vi "plcHMI_scope.vi"() -> ()   [LabVIEW 2020]
doc: "ADS continuos synchronous write example using base blocks. \n\nThe client writes data synchronously and does wait for the respose from server."
uses:
  Agilent/AgilentTotalCluster.ctl
  Agilent/AgilentControl.ctl
  Agilent/Channel Config.ctl
  <vilib>/Platform/TimedLoop/XDataNode/timing_clust.ctl
  <vilib>/Platform/TimedLoop/XDataNode/nitl_modes.ctl
  <vilib>/Platform/TimedLoop/XDataNode/wakeup.ctl
  <vilib>/Platform/TimedLoop/XDataNode/XDataNode.xnode
  <vilib>/Platform/TimedLoop/XDataNode/XDNodeRunTimeDep.lvlib
panel:
  in  "Tab Control":T1(tab)
  in  "Symbol file path - MUST BE ENTERED\nLoad \"ADS Write AND Read Symbols REV X.X.xml\"":path
  in  "EXIT HMI":bool caption="STOP HMI\nEXIT HMI"
  in  "CH4 Vertical Units":string(combo)="V"
  in  "CH4 Vertical Units/div":dbl=2.0
  in  "Toggle Scope Scale":bool
  in  "CH1 Vertical Units/div":dbl=2.0
  in  "CH1 Vertical Units":string(combo)="V"
  in  "Horizontal Units":enum16{"us", "ms", "s"}(ring)
  in  "Horizontal Units/div":dbl=200.0
  out "Download":bool
  in  "Single":bool
  in  "Stop":bool
  in  "Agilent Array":T2[](array[typedef])
  in  "C:\\HVTest\\Local_Cap_Log_Scope (.xlsx)":path
  in  "Process Step":i32
  # "CONFIGURATION"
  # "Press STOP HMI instead of\nLabView Abort Execution"
  # "INPUT VARIABLES - For TDK Lambda 802L\nMust be written to before START"
  # "FAULT STATUSES"
  # "Set to -1 for automated\nfull charge to setpoint"
  # "MANUAL CONTROLS"
  # "Does not record during \"wait\" and appends to data file. Must be named with .xlsx"
  # "HV Switch Configuration"
  # "Records during \"Test Running.\" Must be named with .xlsx"
  # "Control Sys Faults"
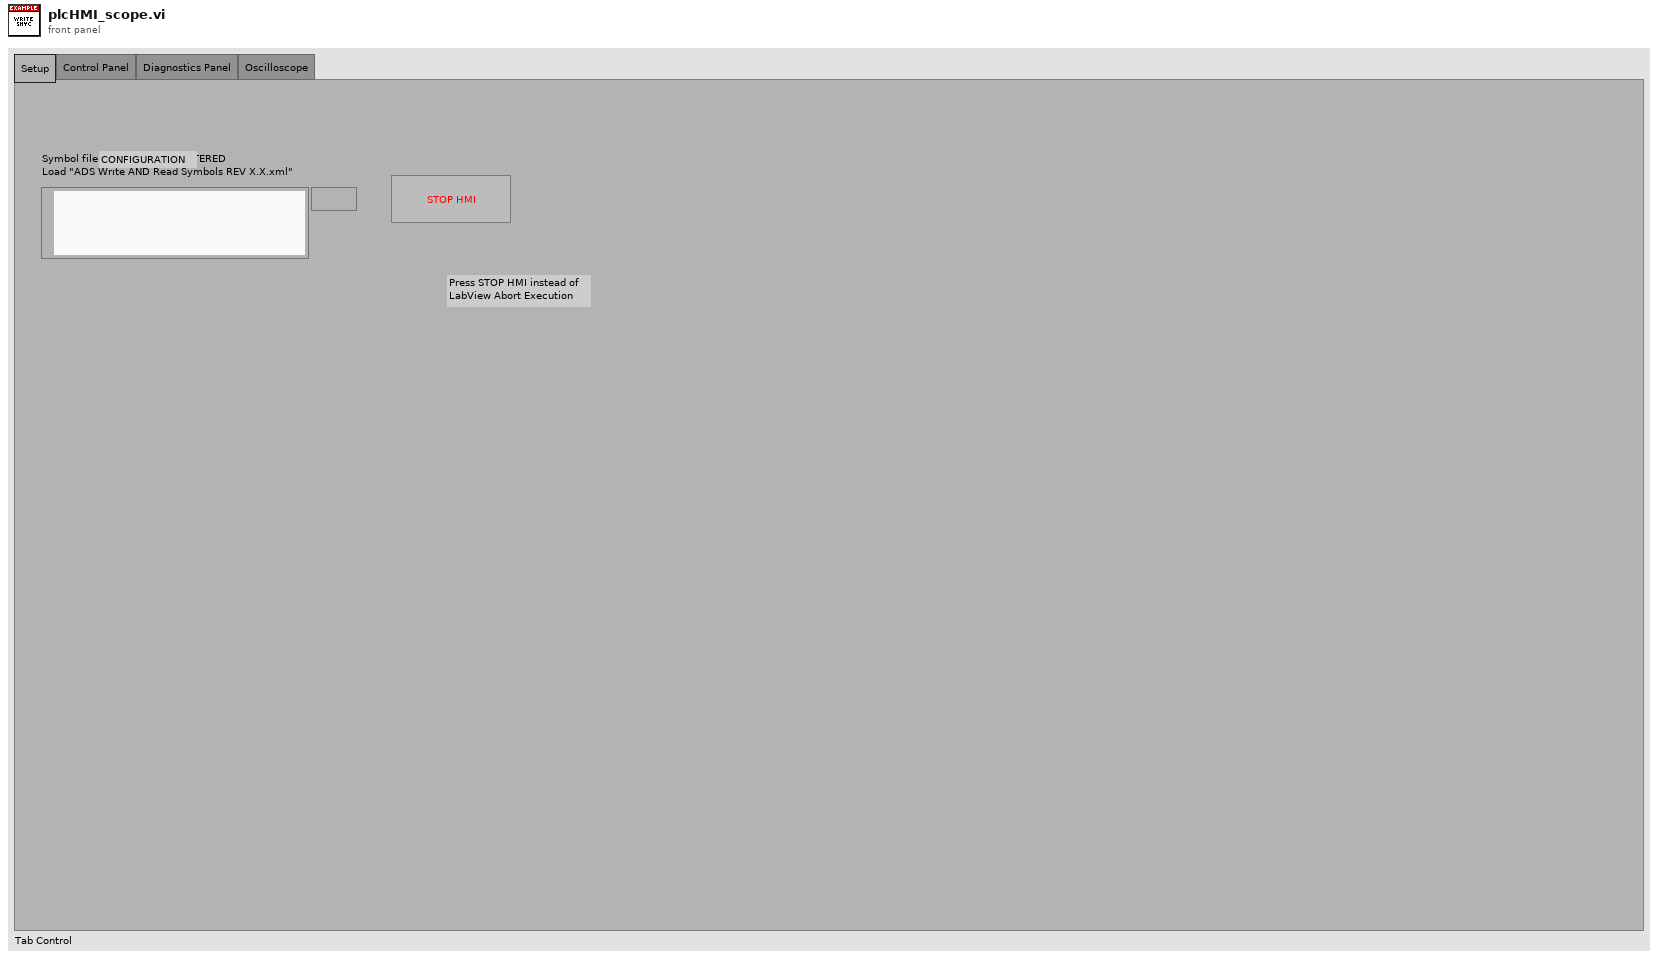
[diagram p1: front panel]
types:
  T1 = enum32{"Setup", "Control Panel", "Diagnostics Panel", "Oscilloscope"}
  T2 = typedef "AgilentTotalCluster.ctl" = cluster{"Agilent Graph":waveform(dbl)[], "Agilent Control":T3, "Agilent Setup Error":errorcluster, "Agilent Present":bool, "Enabled":bool}
  T3 = typedef "AgilentControl.ctl" = cluster{"Trig?":bool, "VISA session":refnum<visa-resource-name>, "Setup to Load":string, "Timeout (ms)":u32, "Desired Samp":enum32{"100", "250", "500", "1000", "2000", "5000", "10000", "20000", "50000", "100000", "200000", "500000", "1000000", "2000000", "4000000", "8000000"}, "Captured Samp":i32, "Desired Channels":T4[]}
  T4 = typedef "Channel Config.ctl" = cluster{"Chan Index":enum16{"Channel1", "Channel2", "Channel3", "Channel4", "MATH"}, "Name":string, "Samples":i32}
  T5 = typedef "XDNodeRunTimeDep.lvlib/timing_clust.ctl" = cluster{"Expected End [f-1]":u64, "Actual End [f-1]":u64, "Finished Late? [f-1]":bool, "Expected End [i-1]":u64, "Actual End [i-1]":u64, "Finished Late? [i-1]":bool, "Expected Start [i]":u64, "Actual Start [i]":u64, "Expected Start [f]":u64, "Actual Start [f]":u64, "Source Name":string, "Structure Name":string, "Period":i64, "Deadline":i64, "Offset":i64, "Start":i64, "Priority":i32, "Timeout":i32, "Mode":T6, "Wakeup Reason":T7, "Error":errorcluster, "Source Type":string, "Secondary Source Type":string, "Global End Time":u64, "Global Start Time":u64, "Frame Duration":u64, "Iteration Duration":u64, "Assigned CPU":i32, "I/O Scan Engine Mode":u32}
  T6 = typedef "XDNodeRunTimeDep.lvlib/nitl_modes.ctl" = enum32{"No Change", "Process missed periods, maintain original phase", "Discard missed periods, maintain original phase", "Process missed periods, ignore original phase", "Discard missed periods, ignore original phase"}
  T7 = typedef "XDNodeRunTimeDep.lvlib/wakeup.ctl" = enum32{"Normal", "Aborted", "Asynchronous wakeup", "Timing source error", "Timed loop error", "Timeout"}
  T8 = cluster{"Agilent Array[0]":T2, "Agilent Array[1]":T2, "Agilent Array[2]":T2, "Agilent Array[3]":T2, "Agilent Array[4]":T2, "Agilent Array[5]":T2, "Agilent Array[6]":T2, "Agilent Array[7]":T2, "Agilent Array[8]":T2}
  T9 = enum32{"100", "250", "500", "1000", "2000", "5000", "10000", "20000", "50000", "100000", "200000", "500000", "1000000", "2000000", "4000000", "8000000"}
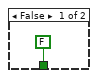
[diagram p2: hidden frame]
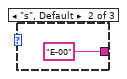
[diagram p5: hidden frame]
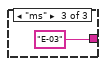
[diagram p6: hidden frame]
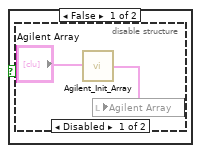
[diagram p7: hidden frame]
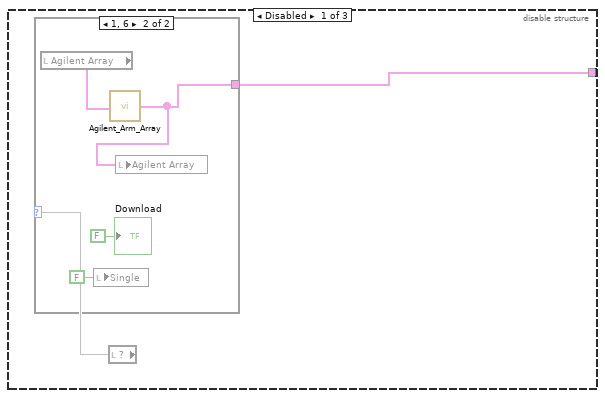
[diagram p11: hidden frame]
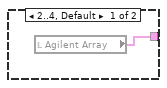
[diagram p12: hidden frame]
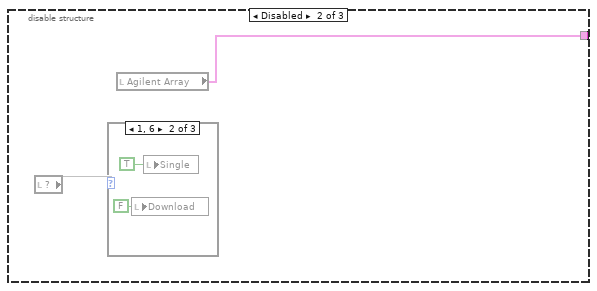
[diagram p13: hidden frame]
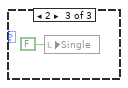
[diagram p15: hidden frame]
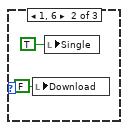
[diagram p17: hidden frame]
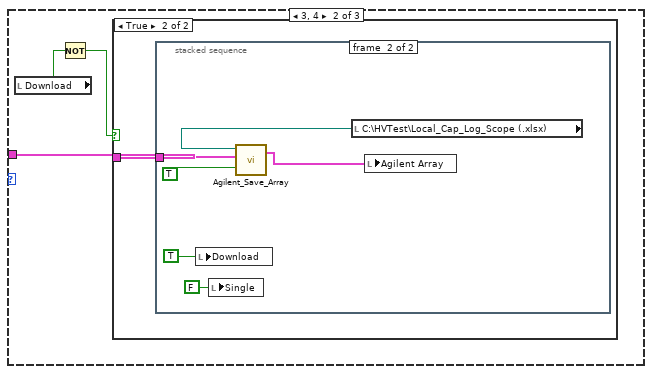
[diagram p19: hidden frame]
diagram:
  # "Symbol Interface"
  n1 = disable-structure shown="Enabled" {
    disable-tunnel: [w5 _] -> _
    disable-tunnel: [w4 w6] -> _
    frame Disabled {
      # "Using Symbol Interface"
      n2 = call <userlib>:"Symbol Interface.vi"() -> ("PortInfo"=w4:string, "error out"=w5:errorcluster)  [unwired: 14 in]
    }
    frame Enabled {
      # "Using Symbol File"
      n3 = Path To String(path="Symbol file path - MUST BE ENTERED\nLoad \"ADS Write AND Read Symbols REV X.X.xml\"") -> (string=w6:string)
    }
  }
  n4 = node-c288(10) -> (w3:T5)  [unwired: 3 in]
  n5 = timed-loop {
    timing: w3 -> [_]
    timing-out: [_] -> w2
    stop <- "EXIT HMI" stop-if-true
    n6 = node-c288() -> ()  [unwired: 1 in, 1 out]
    n7 = disable-structure shown="Enabled" {
      frame Enabled {
        n8 = flat-sequence {
          tunnel: [w65] -> w9
          tunnel: w9 -> [w84]
          frame #0 {
            n9 = disable-structure shown="Enabled" {
              frame Enabled {
                n10 = feedback #1(TRUE) -> (w11:bool)
                n11 = And(x=TRUE, y=w11) -> (x .and. y?=w14:bool)
                n12 = case shown="True" w14 {
                  tunnel: [FALSE FALSE] -> w12
                  frame False {
                  }
                  frame True {
                    n13 = local read "Agilent Array"() -> (w17:T2[])
                    n14 = call "Agilent_Init_Array.vi"("Agilent Array In"=w17) -> ("Agilent Array Out"=w18:T2[])
                    n15 = call "Agilent_Arm_Array.vi"("Agilent Array In"=w18) -> ("Agilent Array Out"=w16:T2[])
                    n16 = local write "Agilent Array"(w16) -> ()
                  }
                }
                n17 = feedback-in #1(w12) -> ()
              }
              frame Disabled {
              }
            }
          }
          frame #1 {
            n18 = case shown="True" "Toggle Scope Scale" {
              frame False {
              }
              frame True {
                n19 = Number To Decimal String(number="CH4 Vertical Units/div") -> (decimal integer string=w24:string)  [unwired: 1 in]
                n20 = Number To Decimal String(number="Horizontal Units/div") -> (decimal integer string=w32:string)  [unwired: 1 in]
                n21 = Number To Decimal String(number="CH1 Vertical Units/div") -> (decimal integer string=w30:string)  [unwired: 1 in]
                n22 = case shown="\"us\"" "Horizontal Units" {
                  tunnel: ["E-06" "E-00" "E-03"] -> w41
                  frame "us" {
                  }
                  frame "s", Default {
                  }
                  frame "ms" {
                  }
                }
                n23 = Concatenate Strings(":CHAN4:SCAL " ("write buffer"), w24, "CH4 Vertical Units") -> (w23:string)
                n24 = Concatenate Strings(":CHAN1:SCAL " ("write buffer"), w30, "CH1 Vertical Units") -> (w37:string)
                n25 = Concatenate Strings(":TIM:SCAL " ("write buffer"), w32, w41) -> (w40:string)
                n26 = VISA Open(VISA resource name=refnum<visa-resource-name> "HV_Test_Scope") -> (VISA resource name=w35:refnum<visa-resource-name>, error out=w36:errorcluster)  [unwired: 4 in]
                n27 = VISA Write(VISA resource name=w35, write buffer=w40, error in (no error)=w36) -> (VISA resource name out=w44:refnum<visa-resource-name>, error out=w43:errorcluster)  [unwired: 1 out]
                n28 = VISA Write(VISA resource name=w44, write buffer=w37, error in (no error)=w43) -> (VISA resource name out=w29:refnum<visa-resource-name>, error out=w27:errorcluster)  [unwired: 1 out]
                n29 = VISA Write(VISA resource name=w29, write buffer=w23, error in (no error)=w27) -> (VISA resource name out=w28:refnum<visa-resource-name>, error out=w26:errorcluster)  [unwired: 1 out]
                n30 = VISA Close(VISA resource name=w28, error in (no error)=w26) -> ()  [unwired: 1 out]
              }
            }
          }
          frame #2 {
            n31 = disable-structure shown="Enabled" {
              frame Enabled {
                n32 = case shown="True" "Stop" {
                  frame False {
                    n33 = disable-structure shown="Disabled" {
                      frame Disabled {
                        n34 = call "Agilent_Init_Array.vi"("Agilent Array In"="Agilent Array") -> ("Agilent Array Out"=w51:T2[])
                        n35 = local write "Agilent Array"(w51) -> ()
                      }
                      frame Enabled {
                      }
                    }
                  }
                  frame True {
                    n36 = VISA Open(VISA resource name=refnum<visa-resource-name> "HV_Test_Scope") -> (VISA resource name=w57:refnum<visa-resource-name>, error out=w58:errorcluster)  [unwired: 4 in]
                    n37 = VISA Write(VISA resource name=w57, write buffer=":STOP", error in (no error)=w58) -> (VISA resource name out=w55:refnum<visa-resource-name>, error out=w56:errorcluster)  [unwired: 1 out]
                    n38 = VISA Close(VISA resource name=w55, error in (no error)=w56) -> ()  [unwired: 1 out]
                  }
                }
              }
              frame Disabled {
              }
            }
            n39 = case shown="True" "Single" {
              frame False {
              }
              frame True {
                n40 = VISA Open(VISA resource name=refnum<visa-resource-name> "HV_Test_Scope") -> (VISA resource name=w63:refnum<visa-resource-name>, error out=w64:errorcluster)  [unwired: 4 in]
                n41 = VISA Write(VISA resource name=w63, write buffer=":SINGLE", error in (no error)=w64) -> (VISA resource name out=w61:refnum<visa-resource-name>, error out=w62:errorcluster)  [unwired: 1 out]
                n42 = VISA Close(VISA resource name=w61, error in (no error)=w62) -> ()  [unwired: 1 out]
              }
            }
          }
          frame #3 {
            n43 = disable-structure shown="Enabled" {
              disable-tunnel: [w67 w74 w79] -> w65
              frame Disabled {
                n44 = local read item#-1() -> (w66)
                n45 = case shown="1, 6" w66 {
                  tunnel: [w68 w72] -> w67
                  frame 2..4, Default {
                    n46 = local read "Agilent Array"() -> (w68:T2[])
                  }
                  frame 1, 6 {
                    n47 = local read "Agilent Array"() -> (w69:T2[])
                    n48 = local write "Single"(FALSE ("Single")) -> ()
                    n49 = call "Agilent_Arm_Array.vi"("Agilent Array In"=w69) -> ("Agilent Array Out"=w72:T2[])
                    n50 = local write "Agilent Array"(w72) -> ()
                    "Download" <- FALSE ("Downloading")
                  }
                }
              }
              frame Disabled {
                n51 = local read item#-1() -> (w73)
                n52 = case shown="1, 6" w73 {
                  frame 0, Default {
                  }
                  frame 1, 6 {
                    n53 = local write "Download"(FALSE ("Download")) -> ()
                    n54 = local write "Single"(TRUE ("Single")) -> ()
                  }
                  frame 2 {
                    n55 = local write "Single"(FALSE ("Single")) -> ()
                  }
                }
                n56 = local read "Agilent Array"() -> (w74:T2[])
              }
              frame Enabled {
                n57 = case shown="2, 7" "Process Step" {
                  frame 0, Default {
                  }
                  frame 1, 6 {
                    n58 = local write "Download"(FALSE ("Download")) -> ()
                    n59 = local write "Single"(TRUE ("Single")) -> ()
                  }
                  frame 2, 7 {
                    n60 = local write "Single"(FALSE ("Single")) -> ()
                  }
                }
                n61 = local read "Agilent Array"() -> (w79:T2[])
              }
            }
          }
          frame #4 {
            n62 = local read "Process Step"() -> (w83:i32)
            n63 = case shown="0" w83 {
              tunnel: w84 -> [_ w87 w100]
              frame Default {
              }
              frame 3, 4 {
                n64 = local read "Download"() -> (w86:bool)
                n65 = Not(x=w86) -> (.not. x?=w85:bool)
                n66 = case shown="True" w85 {
                  tunnel: w87 -> [_ w88]
                  frame False {
                  }
                  frame True {
                    n67 = stacked-sequence {
                      tunnel: w88 -> [_ w98]
                      frame #0 {
                        n68 = local read "Agilent Array"() -> (w92:T2[])
                        n69 = Array To Cluster(array=w92) -> (cluster=w91:T8)
                        n70 = Unbundle By Name(w91) -> ("Agilent Array[0].Agilent Control.Desired Samp"=w89:T9)
                        n71 = call "GF_SetRecordLengthProperly.vi"("Num Samples"=w89, "VISA resource name"=refnum<visa-resource-name> "HV_Test_Scope") -> ()  [unwired: 1 in, 2 out]
                      }
                      frame #1 {
                        n72 = local write "Download"(TRUE ("Downloading")) -> ()
                        n73 = local write "Single"(FALSE ("Single")) -> ()
                        n74 = local read "C:\\HVTest\\Local_Cap_Log_Scope (.xlsx)"() -> (w93:path)
                        n75 = call "Agilent_Save_Array.vi"("Agilent Download"=TRUE, "Agilent Array In"=w98, "File Path"=w93) -> ("Agilent Array Out"=w96:T2[])  [unwired: 1 in, 1 out]
                        n76 = local write "Agilent Array"(w96) -> ()
                      }
                    }
                  }
                }
              }
              frame 0 {
                n77 = local read "Process Step"() -> (w99:i32)
                n78 = case shown="1" w99 {
                  tunnel: w100 -> [_ w103]
                  frame 0, Default {
                  }
                  frame 1 {
                    n79 = local read "Download"() -> (w102:bool)
                    n80 = Not(x=w102) -> (.not. x?=w101:bool)
                    n81 = case shown="True" w101 {
                      tunnel: w103 -> [_ w104]
                      frame False {
                      }
                      frame True {
                        n82 = stacked-sequence {
                          tunnel: w104 -> [_ w114]
                          frame #0 {
                            n83 = local read "Agilent Array"() -> (w108:T2[])
                            n84 = Array To Cluster(array=w108) -> (cluster=w107:T8)
                            n85 = Unbundle By Name(w107) -> ("Agilent Array[0].Agilent Control.Desired Samp"=w105:T9)
                            n86 = call "GF_SetRecordLengthProperly.vi"("Num Samples"=w105, "VISA resource name"=refnum<visa-resource-name> "HV_Test_Scope") -> ()  [unwired: 1 in, 2 out]
                          }
                          frame #1 {
                            n87 = local write "Download"(TRUE ("Downloading")) -> ()
                            n88 = local write "Single"(FALSE ("Single")) -> ()
                            n89 = call "Agilent_Save_Array.vi"("Agilent Download"=TRUE, "Agilent Array In"=w114, "File Path"="C:\\HVTest\\Local_Cap_Log_Scope (.xlsx)") -> ("Agilent Array Out"=w112:T2[])  [unwired: 1 in, 1 out]
                            n90 = local write "Agilent Array"(w112) -> ()
                          }
                        }
                      }
                    }
                  }
                }
              }
            }
          }
        }
      }
      frame Disabled {
      }
    }
    n91 = node-c288() -> ()  [unwired: 1 in, 1 out]
  }
  n92 = node-c288(w2) -> ()  [unwired: 1 out]
